vi "LEP_RV_TestIfWriteSymbol.vi"(8 "Array with names of objects":string[](array[string]), 11 "Symbol's components array":string[](array[string])) -> (3 "Write ?":bool)   [LabVIEW 2011]
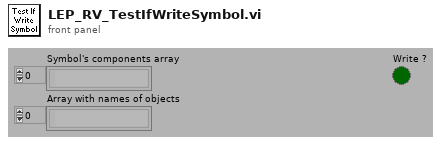
[diagram p1: front panel]
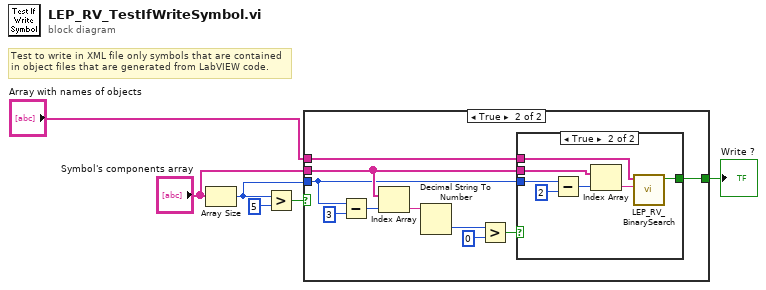
[diagram p0: block diagram]
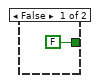
[diagram p2: hidden frame]
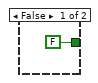
[diagram p3: hidden frame]
diagram:
  # "Test to write in XML file only symbols that are contained in object files that are generated from LabVIEW code."
  n1 = Array Size(array="Symbol's components array") -> (size(s)=w3:i32)
  n2 = Greater?(x=w3, y=5) -> (0:w5:bool)
  n3 = case shown="True" w5 {
    tunnel: "Symbol's components array" -> [_ w11]
    tunnel: w3 -> [_ w10]
    tunnel: [FALSE w8] -> w2
    tunnel: "Array with names of objects" -> [_ w9]
    frame False {
    }
    frame True {
      n4 = Subtract(x=w10, y=3) -> (x-y=w16:i32)
      n5 = Index Array(array=w11, index=w16) -> (element=w15:string)
      n6 = Decimal String To Number(string=w15) -> (number=w14:i32)  [unwired: 2 in, 1 out]
      n7 = Greater?(x=w14, y=0) -> (0:w12:bool)
      n8 = case shown="True" w12 {
        tunnel: w11 -> [_ w25]
        tunnel: w10 -> [_ w24]
        tunnel: w9 -> [_ w21]
        tunnel: [FALSE w19] -> w8
        frame False {
        }
        frame True {
          n9 = Subtract(x=w24, y=2) -> (x-y=w22:i32)
          n10 = Index Array(array=w25, index=w22) -> (element=w20:string)
          n11 = call "LEP_RV_BinarySearch.vi"("x"=w20, "Array"=w21) -> ("Indicate if found x in Array"=w19:bool)  [unwired: 9 in]
        }
      }
    }
  }
  "Write ?" <- w2
